vi "Module Did Init.vi"(8 "error in (no error)":errorcluster, 9 "Initialized?":bool, 10 "Origin":string, 11 "Module ID":i32=-1) -> (0 "error out":errorcluster)   [LabVIEW 2020, in "Camera Acquisition.lvlib"]
doc: "Send the Module Did Init event to any VI registered to listen to this module's broadcast events.\n_____\nBased on DQMH Project Template 6.0.0.91."
uses:
  Camera Acquisition.lvlib
  Did Init Argument--cluster.ctl
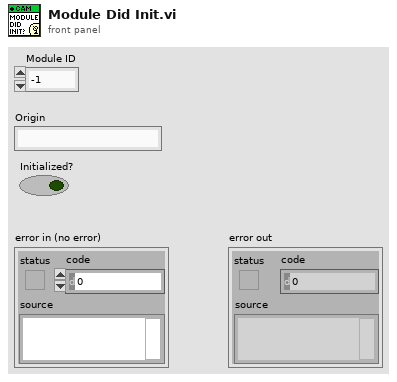
[diagram p1: front panel]
types:
  T1 = typedef "Camera Acquisition.lvlib/Did Init Argument--cluster.ctl" = cluster{"Init?":bool, "Info":string, "Module ID":i32}
  T2 = typedef "Camera Acquisition.lvlib/Broadcast Events--cluster.ctl" = cluster{"Module Did Init":refnum<user-event>, "Status Updated":refnum<user-event>, "Error Reported":refnum<user-event>, "Module Did Stop":refnum<user-event>, "Update Module Execution Status":refnum<user-event>}
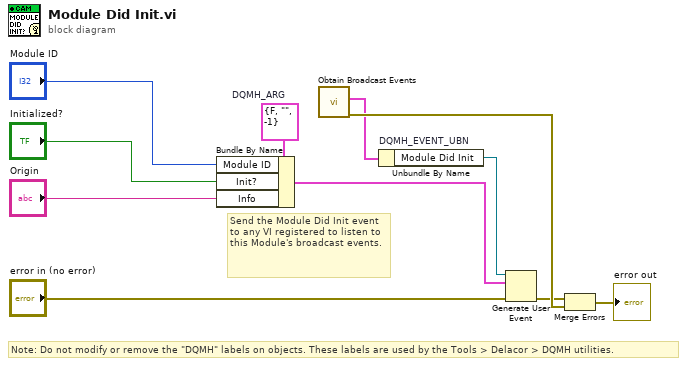
[diagram p0: block diagram]
diagram:
  w3 = T1 {"Init?"=FALSE, "Info"="", "Module ID"=-1}  # DQMH_ARG
  # "Note: Do not modify or remove the \"DQMH\" labels on objects. These labels are used by the Tools > Delacor > DQMH utilities."
  # "Send the Module Did Init event to any VI registered to listen to this Module's broadcast events."
  n1 = Bundle By Name(cluster=w3, "Module ID"="Module ID", "Init?"="Initialized?", "Info"="Origin") -> (w2:T1)
  n2 = call "Obtain Broadcast Events.vi"() -> ("error out"=w7:errorcluster, "Camera Acquisition Broadcast Events"=w5:T2)  [unwired: 10 in]
  n3 = Unbundle By Name "DQMH_EVENT_UBN"(w5) -> ("Module Did Init"=w4:refnum<user-event>)
  n4 = Generate User Event(user event=w4, event data cluster=w2, error in="error in (no error)") -> (error out=w6:errorcluster)  [unwired: 1 in, 1 out]
  n5 = Merge Errors(w6, w7) -> (→"error out":errorcluster)
